vi "parse_spec-data.vi"(11 "String":string="00.00.00.00.00.00.00.00.00.00.00.00.00.00.00.00.00.00.00.00.%\n") -> (0 "Array 2":u16[](array[numeric]))   [LabVIEW 2020]
panel:
  out "deleted portion":string[](array[string])=["%\n"]
  out "Array":string[](array[string])=["00", "00", "00", "00", "00", "00", "00", "00", "00", "00", "00", "00", "00", "00", "00", "00", "00", "00", "00", "00"]
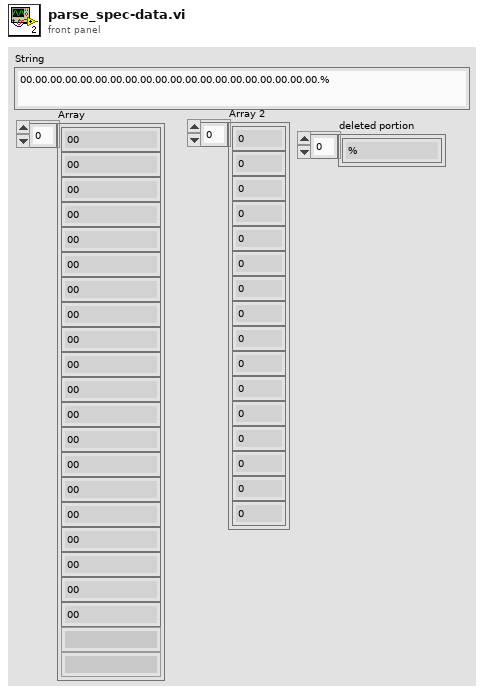
[diagram p1: front panel]
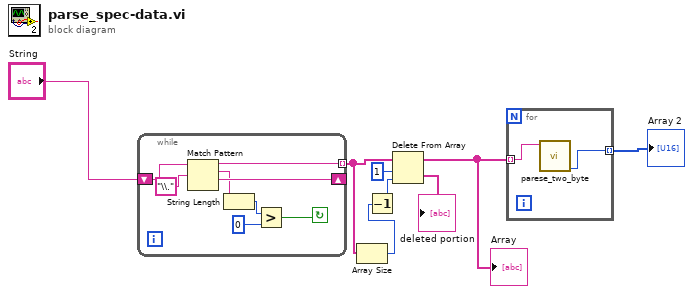
[diagram p0: block diagram]
diagram:
  n1 = while {
    tunnel: [w16] -> w5 mode=indexing
    shift-right: [w14] -> _
    shift-left: "String" -> [w13]
    stop <- w9 continue-if-true
    n2 = Match Pattern(string=w13, regular expression="\\.") -> (before substring=w16:string, match substring=w10:string, after substring=w14:string)  [unwired: 1 in, 1 out]
    n3 = String Length(string=w10) -> (length=w11:i32)
    n4 = Greater?(x=w11, y=0) -> (0:w9:bool)
  }
  n5 = Array Size(array=w5) -> (size(s)=w4:i32)
  n6 = Decrement(x=w4) -> (x-1=w3:i32)
  n7 = Delete From Array(array=w5, length=1, index=w3) -> (deleted portion=→"deleted portion":string[], array with subset deleted=w1:string[])
  "Array" <- w1
  n8 = for {
    tunnel: w1 -> [w18] mode=indexing
    tunnel: [w17] -> w2 mode=indexing
    n9 = call "parese_two_byte.vi"("write buffer 2"=w18) -> ("x+y"=w17:u16)  [unwired: 10 in]
  }
  "Array 2" <- w2
